vi "user32_DrawCaption.vi"(0 "hWnd":u32, 1 "uFlags":u32(ring) items=["DC_ACTIVE"=1, "DC_SMALLCAP"=2, "DC_ICON"=4, "DC_TEXT"=8, "DC_INBUTTON"=16, "DC_GRADIENT"=32, "DC_BUTTONS"=64], 5 "hdc":u32, 7 "Rect":T1, 11 "错误输入（无错误）":errorcluster) -> (4 "dup hWnd":u32, 6 "success?":bool, 15 "错误输出":errorcluster)   [LabVIEW 2011]
doc: "该函数绘制窗口标题栏。\n\n绘制选项，该参数可以是一个或多个以下值之一：\nDC_ACTIVE 使用活动标题栏颜色；\nDC_SMALLCAP 使用当前小标题栏字体；\nDC_ICON 使用图标；\nDC_TEXT 绘制标题；\nDC_INBUTTON 按下状态；\nDC_GRADIENT 使用渐变色；\nDC_BUTTONS 如果设置，在标题栏上绘制按钮（按照应用程序的最小化、还原或关闭按钮）。"
uses:
  user32.dll
panel:
  # "参数BUTTON值未确定"
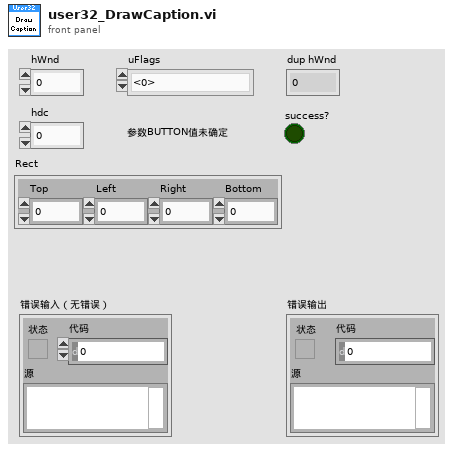
[diagram p1: front panel]
types:
  T1 = cluster{"Top":i32, "Left":i32, "Right":i32, "Bottom":i32}
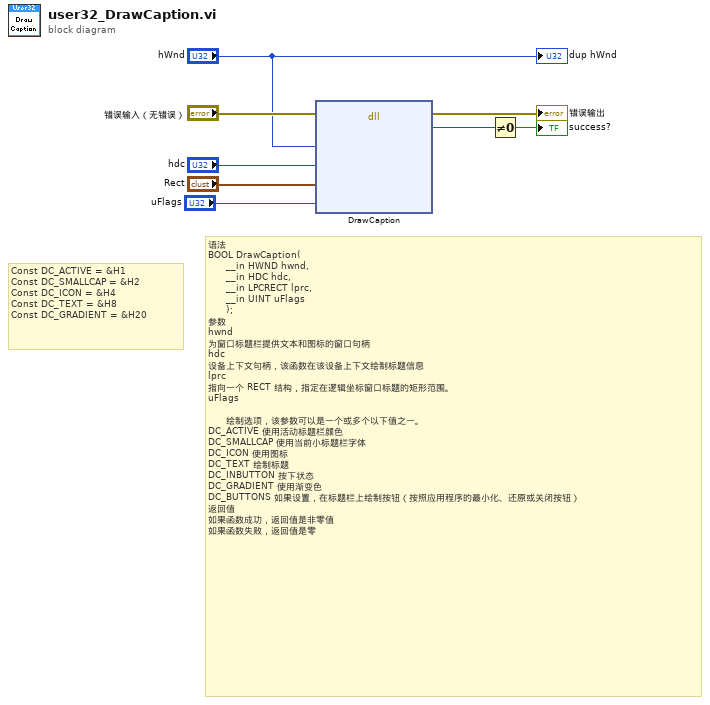
[diagram p0: block diagram]
diagram:
  # "Const DC_ACTIVE = &H1\nConst DC_SMALLCAP = &H2\nConst DC_ICON = &H4\nConst DC_TEXT = &H8\nConst DC_GRADIENT = &H20"
  # "语法\nBOOL DrawCaption(\n　　__in HWND hwnd,\n　　__in HDC hdc,\n　　__in LPCRECT lprc,\n　　__in UINT uFlags\n　　);\n参数\nhwnd\n为窗口标题栏提供文本和图标的窗口句柄\nhdc\n设备上下文句柄，该函数在该设备上下文绘制标题信息\nlprc\n指向一个 RECT 结构，指定在逻辑坐标窗口标题的矩形范围。\nuFlags\n　　\n　　绘制选项，该参数可以是一个或多个以下值之一。\nDC_ACTIVE 使用活动标题栏颜色\nDC_SMALLCAP 使用当前小标题栏字体\nDC_ICON 使用图标\nDC_TEXT 绘制标题\nDC_INBUTTON 按下状态\nDC_GRADIENT 使用渐变色\nDC_BUTTONS 如果设置，在标题栏上绘制按钮（按照应用程序的最小化、还原或关闭按钮）\n返回值\n如果函数成功，返回值是非零值\n如果函数失败，返回值是零"
  n1 = dll-call lib="user32.dll" fn="DrawCaption"(error in="错误输入（无错误）", "hWnd"="hWnd", "hdc"="hdc", "lprc"="Rect", "uFlags"="uFlags") -> (error out=→"错误输出":errorcluster, "Bool"=w5:u8)  [unwired: 6 in, 1 out]
  n2 = Not Equal To 0?(x=w5) -> (x != 0?=→"success?":bool)
  "dup hWnd" <- "hWnd"
